vi "Replace negative values from 2d array.vi"() -> ()   [LabVIEW 2017]
panel:
  out "coerced(x)":dbl[][](array[numeric])
  out "In Range?":bool[][](array[boolean])
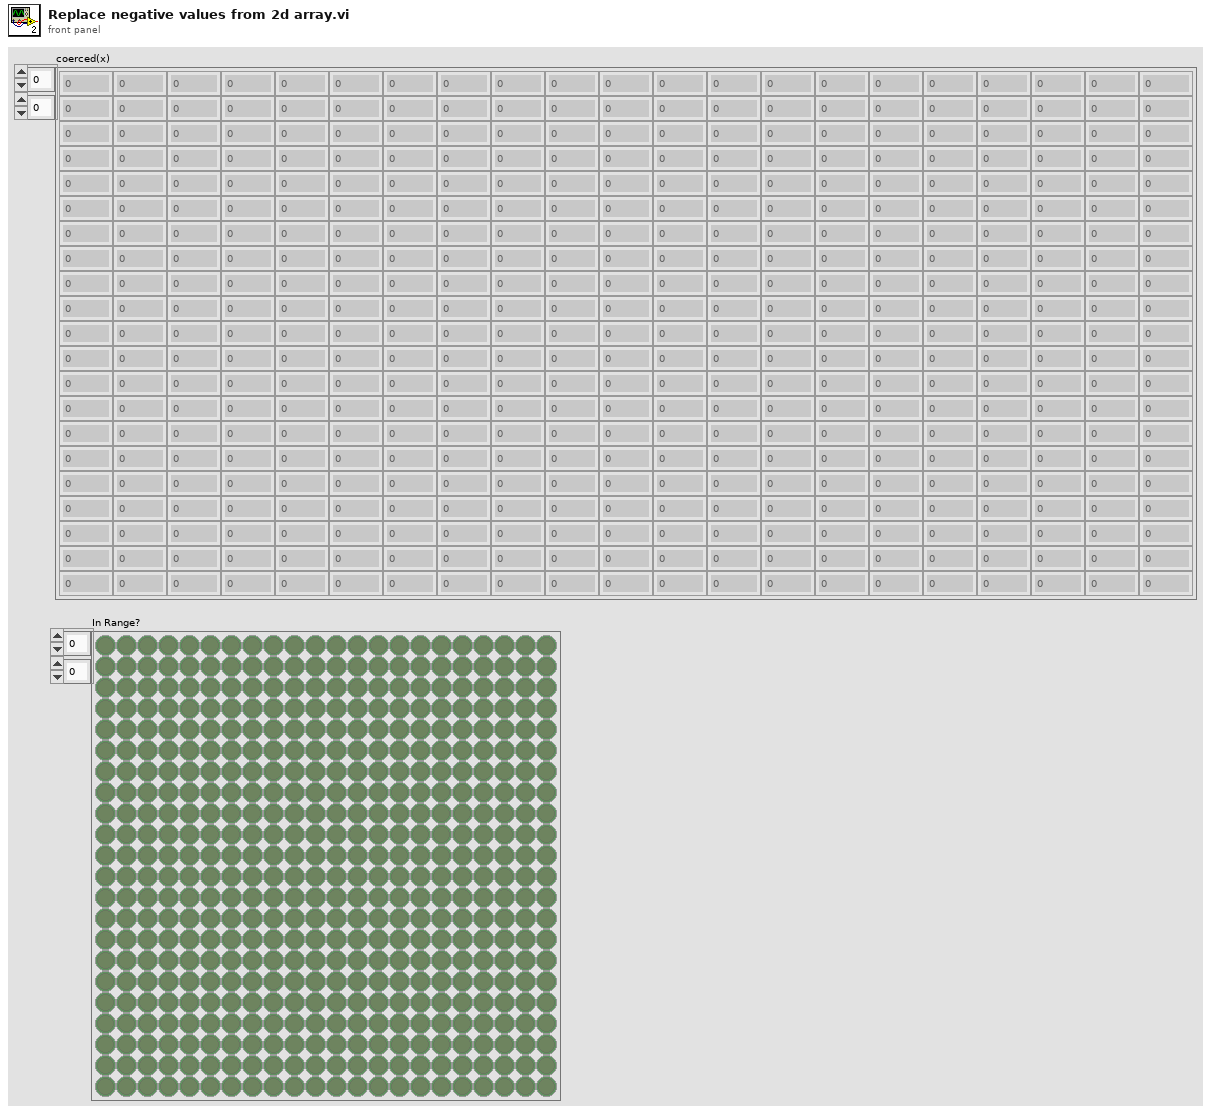
[diagram p1: front panel]
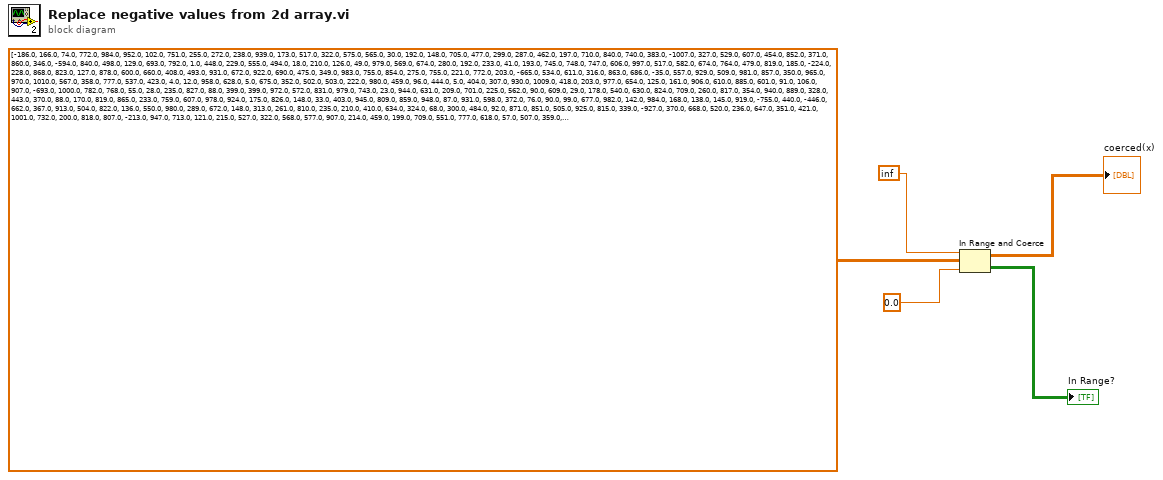
[diagram p0: block diagram]
diagram:
  n1 = In Range and Coerce(upper limit=inf, x=dbl[][] [[-186.0, 166.0, 74.0, 772.0, 984.0, 952.0, 102.0, 751.0, 255.0, 272.0, 238.0, 939.0, 173.0, 517.0, 322.0, 575.0, 565.0, 30.0, 192.0, 148.0], [705.0, 477.0, 299.0, 287.0, 462.0, 197.0, 710.0, 840.0, 740.0, 383.0, -1007.0, 327.0, 529.0, 607.0, 454.0, 852.0, 371.0, 860.0, 346.0, -594.0], [840.0, 498.0, 129.0, 693.0, 792.0, 1.0, 448.0, 229.0, 555.0, 494.0, 18.0, 210.0, 126.0, 49.0, 979.0, 569.0, 674.0, 280.0, 192.0, 233.0], [41.0, 193.0, 745.0, 748.0, 747.0, 606.0, 997.0, 517.0, 582.0, 674.0, 764.0, 479.0, 819.0, 185.0, -224.0, 228.0, 868.0, 823.0, 127.0, 878.0], [600.0, 660.0, 408.0, 493.0, 931.0, 672.0, 922.0, 690.0, 475.0, 349.0, 983.0, 755.0, 854.0, 275.0, 755.0, 221.0, 772.0, 203.0, -665.0, 534.0], [611.0, 316.0, 863.0, 686.0, -35.0, 557.0, 929.0, 509.0, 981.0, 857.0, 350.0, 965.0, 970.0, 1010.0, 567.0, 358.0, 777.0, 537.0, 423.0, 4.0], [12.0, 958.0, 628.0, 5.0, 675.0, 352.0, 502.0, 503.0, 222.0, 980.0, 459.0, 96.0, 444.0, 5.0, 404.0, 307.0, 930.0, 1009.0, 418.0, 203.0], [977.0, 654.0, 125.0, 161.0, 906.0, 610.0, 885.0, 601.0, 91.0, 106.0, 907.0, -693.0, 1000.0, 782.0, 768.0, 55.0, 28.0, 235.0, 827.0, 88.0], [399.0, 399.0, 972.0, 572.0, 831.0, 979.0, 743.0, 23.0, 944.0, 631.0, 209.0, 701.0, 225.0, 562.0, 90.0, 609.0, 29.0, 178.0, 540.0, 630.0], [824.0, 709.0, 260.0, 817.0, 354.0, 940.0, 889.0, 328.0, 443.0, 370.0, 88.0, 170.0, 819.0, 865.0, 233.0, 759.0, 607.0, 978.0, 924.0, 175.0], [826.0, 148.0, 33.0, 403.0, 945.0, 809.0, 859.0, 948.0, 87.0, 931.0, 598.0, 372.0, 76.0, 90.0, 99.0, 677.0, 982.0, 142.0, 984.0, 168.0], [138.0, 145.0, 919.0, -755.0, 440.0, -446.0, 662.0, 367.0, 913.0, 504.0, 822.0, 136.0, 550.0, 980.0, 289.0, 672.0, 148.0, 313.0, 261.0, 810.0], [235.0, 210.0, 410.0, 634.0, 324.0, 68.0, 300.0, 484.0, 92.0, 871.0, 851.0, 505.0, 925.0, 815.0, 339.0, -927.0, 370.0, 668.0, 520.0, 236.0], [647.0, 351.0, 421.0, 1001.0, 732.0, 200.0, 818.0, 807.0, -213.0, 947.0, 713.0, 121.0, 215.0, 527.0, 322.0, 568.0, 577.0, 907.0, 214.0, 459.0], [199.0, 709.0, 551.0, 777.0, 618.0, 57.0, 507.0, 359.0, 797.0, 113.0, 128.0, 623.0, 839.0, 434.0, 1003.0, 247.0, 382.0, 75.0, 314.0, 716.0], [969.0, 289.0, 655.0, 676.0, 942.0, 440.0, 870.0, 196.0, 926.0, 101.0, 495.0, 878.0, 843.0, 394.0, 160.0, 149.0, 678.0, 7.0, 471.0, 164.0], [552.0, 571.0, 431.0, 661.0, 584.0, 91.0, 386.0, 393.0, 1022.0, 259.0, 472.0, 849.0, 478.0, 166.0, 178.0, 870.0, 780.0, 673.0, 923.0, 102.0], [589.0, -308.0, 906.0, 769.0, 880.0, 35.0, 863.0, 563.0, 33.0, 594.0, 10.0, 311.0, 140.0, 314.0, 47.0, 178.0, 519.0, 638.0, 435.0, 790.0], [636.0, 236.0, 501.0, 406.0, 883.0, 317.0, 922.0, 143.0, 261.0, 493.0, 122.0, 178.0, 53.0, 574.0, 705.0, 763.0, 214.0, 268.0, 1006.0, 866.0], [114.0, 195.0, 318.0, 135.0, 919.0, 730.0, 158.0, 617.0, 310.0, 442.0, 524.0, 510.0, 671.0, 1005.0, 350.0, 721.0, 998.0, 740.0, 932.0, 212.0]] ("Array after"), lower limit=0.0) -> (coerced(x)=→"coerced(x)":dbl[][], In Range?=→"In Range?":bool[][])
